vi "toadd.vi"   [LabVIEW 2021]
uses:
  globalvariables.vi
types:
  T1 = cluster{"Control Sensor Offset":dbl, "Set Limit Low":dbl, "Set Limit High":dbl, "Derivative Gain":dbl, "Integral Gain":dbl, "Proportional Bandwidth":dbl}
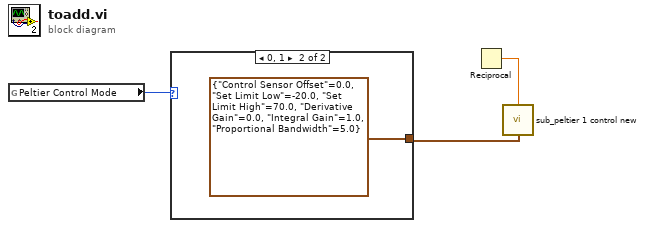
[diagram p0: block diagram]
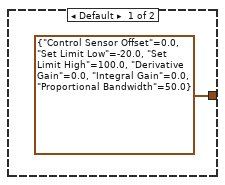
[diagram p2: hidden frame]
diagram:
  n1 = global read "globalvariables.vi" "Peltier Control Mode"() -> (w3:i16)
  n2 = case shown="0, 1" w3 {
    tunnel: [T1 {"Control Sensor Offset"=0.0, "Set Limit Low"=-20.0, "Set Limit High"=100.0, "Derivative Gain"=0.0, "Integral Gain"=0.0, "Proportional Bandwidth"=50.0} ("Control Settings") T1 {"Control Sensor Offset"=0.0, "Set Limit Low"=-20.0, "Set Limit High"=70.0, "Derivative Gain"=0.0, "Integral Gain"=1.0, "Proportional Bandwidth"=5.0} ("Control Settings")] -> w2
    frame Default {
    }
    frame 0, 1 {
    }
  }
  n3 = Reciprocal() -> (1/x=w1:dbl)  [unwired: 1 in]
  n4 = call "sub_peltier 1 control new.vi"("Sample Rate (s)"=w1, "Control Settings"=w2) -> ()  [unwired: 14 in]
